vi "BestYForAnyElements.vi"(8 "inimigos":bool=TRUE, 9 "Position to be analyzed":dbl[](array[numeric]), 10 "Game":refnum<class "Game.lvclass">, 11 "Utilities in":refnum<class "Utilities.lvclass">) -> (2 "Goal Gap":dbl, 3 "Utilities out":refnum<class "Utilities.lvclass">)   [LabVIEW 2023, in "Utilities.lvclass"]
uses:
  Utilities.lvclass
  segment.ctl
  Game_class/Game.lvclass
  Vision_class/Old vision/SSL Detection Frame Simple Estimator Cameras VelCmd Folder/Core/AI Ball.ctl
  pos.ctl
  Game_class/Game.lvclass/Game.ctl
  Team_class/Team.lvclass/Team.ctl
  Object_class/Object.lvclass/Object.ctl
  Object_class/Read x.vi
  Object_class/Read y.vi
  <vilib>/Analysis/baseanly.llb/Real Dot Product.vi
  Game_class/Read FieldRef.vi
  Game_class/Read EnemyRef.vi
  Game_class/Read AllyRef.vi
  Team_class/Read RobotRef.vi
  Ally_class/Ally.lvclass
  C:/Users/roboi/Downloads/VSS_AI-Larc2023 - Copia (2)/Team_class/Team.lvclass
  Enemy_class/Enemy.lvclass
  Robot_class/Robot.lvclass
  C:/Users/roboi/Downloads/VSS_AI-Larc2023 - Copia (2)/Object_class/Object.lvclass
  Field_class/Field.lvclass
  <vilib>/Analysis/NI_AALBase.lvlib
panel:
  out "Best y":dbl
  out "Gap Coord":dbl[](array[numeric])
  in  "eclipse angle eps":dbl=0.035 format="%#_13g"
  out "Eclipse":bool
  out "Vetor de segmentos (sombras)":T1[](array[typedef])
  out "Vetor de segmentos ordenado":T1[](array[typedef])
  out "pilha output (merged)":T1[](array[typedef])
  in  "Maior intervalo":bool
  out "Vetor de gaps":T1[](array[typedef])
  in  "Best y para varredura?":bool
  in  "Ball false":dbl[](array[numeric])
  out "Vetor de gaps \ncorreto":T1[](array[typedef])
  out "error out":errorcluster
  in  "error in (no error)":errorcluster
types:
  T1 = typedef "Utilities.lvclass/segment.ctl" = cluster{"up":dbl, "down":dbl}
  T2 = typedef "pos.ctl" = cluster{"x":dbl, "y":dbl}
  T3 = typedef "AI Ball.ctl" = cluster{"x":dbl, "y":dbl, "timestamp":timestamp, "Vel_x":dbl, "Vel_y":dbl, "Pos Bola Est":dbl[], "Valid":bool}
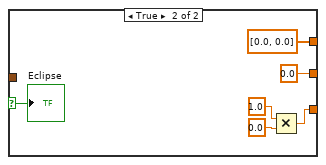
[diagram p4: hidden frame]
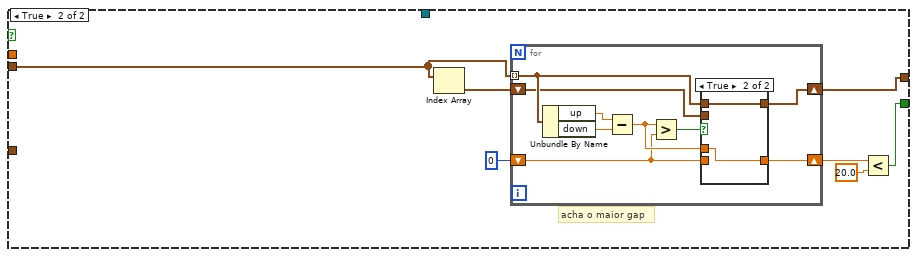
[diagram p7: hidden frame]
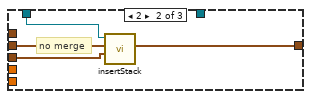
[diagram p9: hidden frame]
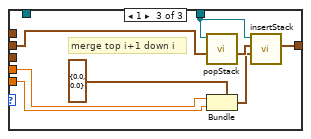
[diagram p10: hidden frame]
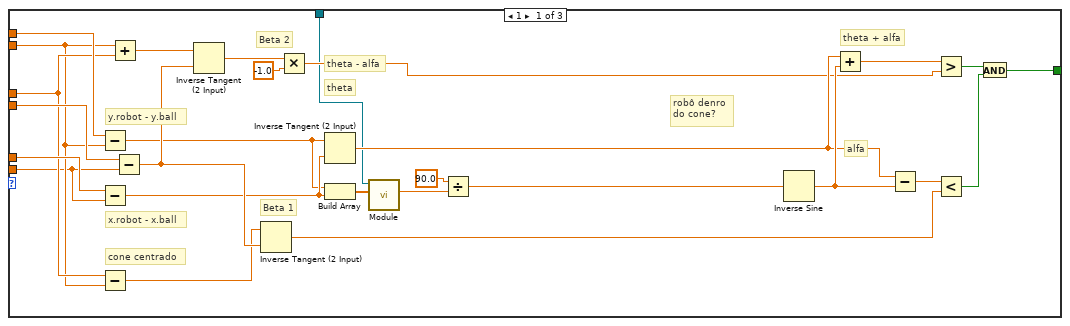
[diagram p12: hidden frame]
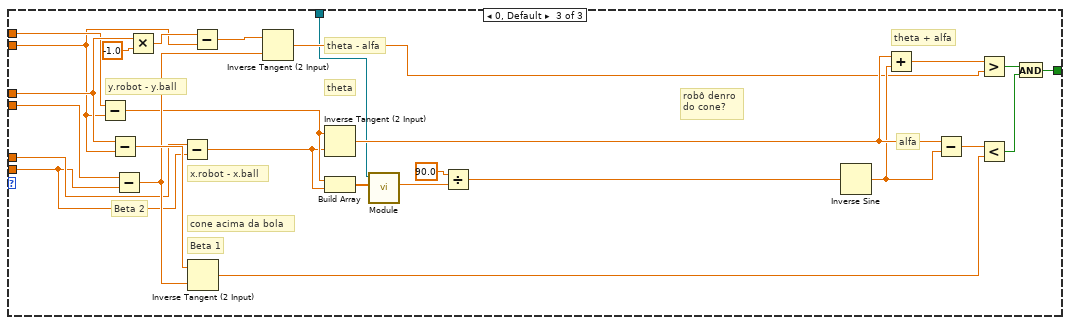
[diagram p13: hidden frame]
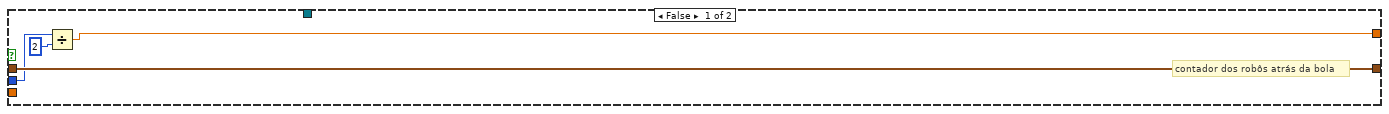
[diagram p14: hidden frame]
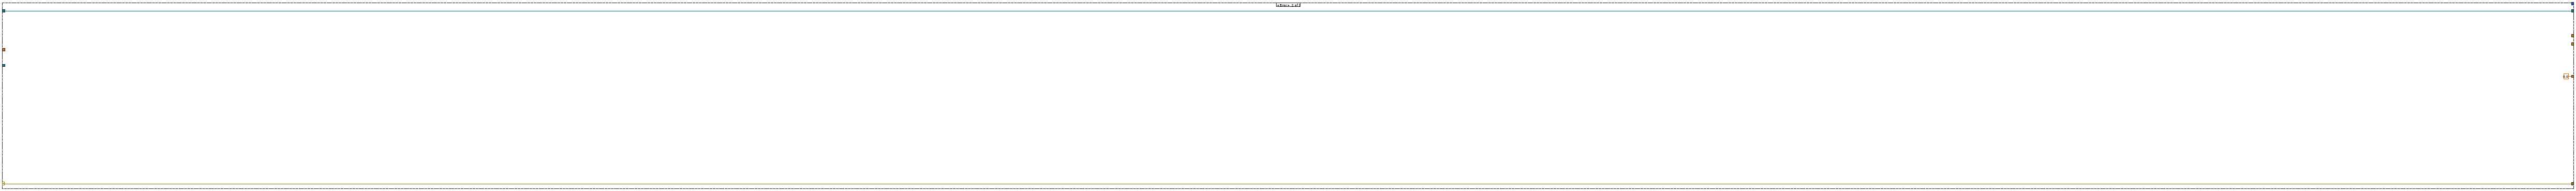
[diagram p16: hidden frame]
diagram:
  # "Gap kick is now a value from 0 to 1\n0 -> goal not free\n1 - > goal totally free"
  n1 = case shown="No Error" "error in (no error)" {
    selector: "error in (no error)" -> [w64 w427]
    tunnel: [w64 w427] -> w10
    tunnel: [w17 w426] -> w8
    tunnel: "Utilities in" -> [w17 w426]
    tunnel: "Game" -> [w29 _]
    tunnel: [w28 _] -> w6
    tunnel: [w27 _] -> w2
    tunnel: [w26 0.0] -> w5
    tunnel: [w16 _] -> w3
    tunnel: "Position to be analyzed" -> [w15 _]
    frame No Error {
      w42 = T3 {"x"=0.0, "y"=0.0, "timestamp"=timestamp(0 s since 1904-01-01), "Vel_x"=0.0, "Vel_y"=0.0, "Pos Bola Est"=[], "Valid"=FALSE} ("element")
      # "goal_width/2"
      # "field_length/2"
      # "balls"
      # "vetor de gaps"
      # "upper"
      n2 = property class="Game"(reference=w29) -> ("FieldRef"=w24:refnum<class "Field.lvclass">, "EnemyRef"=w21:refnum<class "Enemy.lvclass">, "AllyRef"=w19:refnum<class "Ally.lvclass">)  [unwired: 1 in, 2 out]
      n3 = property class="Enemy"(reference=w21) -> ("RobotRef"=w20:refnum<class "Robot.lvclass">[])  [unwired: 1 in, 2 out]
      n4 = property class="Ally"(reference=w19) -> ("RobotRef"=w18:refnum<class "Robot.lvclass">[])  [unwired: 1 in, 2 out]
      n5 = Index Array(array=w15) -> (element #1=w14:dbl, element #2=w13:dbl)  [unwired: 2 in]
      n6 = property class="Field"(reference=w24) -> ("field_length"=w22:i32, "goal_width"=w16:i32)  [unwired: 1 in, 2 out]
      n7 = Bundle By Name(cluster=T2 {"x"=0.0, "y"=0.0} ("pos"), "x"=w14, "y"=w13) -> (w23:T2)
      n8 = Select(t=w20, s="inimigos", f=w18) -> (s? t:f=w46:refnum<class "Robot.lvclass">[])
      n9 = Index Array(array="Ball false") -> (element #1=w45:dbl, element #2=w44:dbl)  [unwired: 2 in]
      n10 = Bundle By Name(cluster=w42, "x"=w45, "y"=w44) -> ()  [unwired: 1 out]
      n11 = case shown="False" "Best y para varredura?" {
        tunnel: [w119 w120] -> w41
        tunnel: w23 -> [w119 w120]
        tunnel: w42 -> [_ _]
        frame False {
        }
        frame True {
        }
      }
      n12 = Divide(x=w16, y=u32 2 ("x")) -> (x/y=w34:dbl)
      n13 = for {
        shift-right: [w268] -> w49
        shift-left: T1[] [] -> [w267]
        tunnel: w22 -> [w245]
        tunnel: w34 -> [w247]
        tunnel: w34 -> [w265]
        shift-right: [w264] -> w47
        shift-left: _ -> [_]
        tunnel: w46 -> [w237] mode=indexing
        tunnel: "inimigos" -> [w262]
        tunnel: w41 -> [w241]
        tunnel: w17 -> [w234]
        tunnel: w17 -> [w233]
        # "y ball"
        # "x ball"
        # "y.robot"
        # "x.robot"
        # "field_length/2"
        # "goal_width/2"
        # "y ball"
        # "x ball"
        n14 = property class="Robot"(reference=w237) -> ("x"=w236:dbl, "y"=w235:dbl)  [unwired: 1 in, 2 out]
        n15 = Unbundle By Name(w241) -> ("x"=w240:dbl, "y"=w238:dbl)
        n16 = Divide(x=w245, y=2.0) -> (x/y=w244:dbl)
        n17 = Multiply(x=w247, y=-1.0) -> (x*y=w251:dbl)
        n18 = Greater?(x=w238, y=w247) -> (0:w250:bool)
        n19 = Less?(x=w238, y=w251) -> (x < y?=w249:bool)
        n20 = Absolute Value(x=w240) -> (abs(x)=w260:dbl)
        n21 = Absolute Value(x=w236) -> (abs(x)=w266:dbl)
        n22 = Multiply(x=w236, y=-1.0) -> (x*y=w261:dbl)
        n23 = Greater?(x=w266, y=w260) -> (0:w259:bool)
        n24 = Select(t=w236, s=w262, f=w261) -> (s? t:f=w242:dbl)
        n25 = Select(t=1, s=w250, f=0) -> (s? t:f=w257:i32)
        n26 = Select(t=0, s=w249, f=1) -> (s? t:f=w258:i32)
        n27 = Add(x=w257, y=w258) -> (x+y=w248:i32)
        n28 = case shown="2" w248 {
          tunnel: w247 -> [w272 w299 w348]
          tunnel: w244 -> [w293 w319 w350]
          tunnel: w242 -> [w280 w306 w343]
          tunnel: w235 -> [w279 w307 w344]
          tunnel: [w281 w308 w334] -> w239
          tunnel: w240 -> [w270 w297 w326]
          tunnel: w238 -> [w271 w298 w327]
          tunnel: w234 -> [w269 w296 w325]
          frame 1 {
            # "robô denro\ndo cone?"
            # "cone centrado"
            # "theta - alfa"
            # "theta + alfa"
            # "theta"
            # "alfa"
            # "x.robot - x.ball"
            # "y.robot - y.ball"
            # "Beta 2"
            # "Beta 1"
            n29 = Subtract(x=w279, y=w271) -> (x-y=w282:dbl)
            n30 = Subtract(x=w280, y=w270) -> (x-y=w283:dbl)
            n31 = Subtract(x=w272, y=w271) -> (x-y=w294:dbl)
            n32 = Add(x=w271, y=w272) -> (x+y=w292:dbl)
            n33 = Subtract(x=w293, y=w270) -> (x-y=w295:dbl)
            n34 = Inverse Tangent (2 Input)(1:w295, 2:w292) -> (0:w291:dbl)
            n35 = Inverse Tangent (2 Input)(1:w295, 2:w294) -> (0:w275:dbl)
            n36 = Multiply(x=w291, y=-1.0) -> (x*y=w277:dbl)
            n37 = Inverse Tangent (2 Input)(1:w283, 2:w282) -> (0:w288:dbl)
            n38 = Build Array(w282, w283) -> (w284:dbl[])
            n39 = call "Module.vi"("2D vector"=w284, "Utilities in"=w269) -> ("Modulo"=w285:dbl)  [unwired: 7 in, 2 out]
            n40 = Divide(x=90.0, y=w285) -> (x/y=w286:dbl)
            n41 = Inverse Sine(1:w286) -> (0:w289:dbl)
            n42 = Add(x=w288, y=w289) -> (x+y=w278:dbl)
            n43 = Subtract(x=w288, y=w289) -> (x-y=w276:dbl)
            n44 = Greater?(x=w278, y=w277) -> (0:w273:bool)
            n45 = Less?(x=w276, y=w275) -> (x < y?=w274:bool)
            n46 = And(x=w273, y=w274) -> (x .and. y?=w281:bool)
          }
          frame 2 {
            # "robô denro\ndo cone?"
            # "cone abaixo da bola"
            # "theta - alfa"
            # "theta + alfa"
            # "theta"
            # "alfa"
            # "x.robot - x.ball"
            # "y.robot - y.ball"
            # "Beta 2"
            # "Beta 1"
            n47 = Add(x=w298, y=w299) -> (x+y=w322:dbl)
            n48 = Subtract(x=w298, y=w299) -> (x-y=w321:dbl)
            n49 = Subtract(x=w319, y=w297) -> (x-y=w320:dbl)
            n50 = Inverse Tangent (2 Input)(1:w320, 2:w321) -> (0:w317:dbl)
            n51 = Inverse Tangent (2 Input)(1:w320, 2:w322) -> (0:w323:dbl)
            n52 = Subtract(x=w307, y=w298) -> (x-y=w309:dbl)
            n53 = Multiply(x=w323, y=-1.0) -> (x*y=w304:dbl)
            n54 = Subtract(x=w306, y=w297) -> (x-y=w310:dbl)
            n55 = Inverse Tangent (2 Input)(1:w310, 2:w309) -> (0:w315:dbl)
            n56 = Build Array(w309, w310) -> (w311:dbl[])
            n57 = call "Module.vi"("2D vector"=w311, "Utilities in"=w296) -> ("Modulo"=w312:dbl)  [unwired: 7 in, 2 out]
            n58 = Multiply(x=w317, y=-1.0) -> (x*y=w302:dbl)
            n59 = Divide(x=90.0, y=w312) -> (x/y=w313:dbl)
            n60 = Inverse Sine(1:w313) -> (0:w316:dbl)
            n61 = Add(x=w315, y=w316) -> (x+y=w305:dbl)
            n62 = Subtract(x=w315, y=w316) -> (x-y=w303:dbl)
            n63 = Less?(x=w303, y=w302) -> (x < y?=w301:bool)
            n64 = Greater?(x=w305, y=w304) -> (0:w300:bool)
            n65 = And(x=w300, y=w301) -> (x .and. y?=w308:bool)
          }
          frame 0, Default {
            # "robô denro\ndo cone?"
            # "cone acima da bola"
            # "theta - alfa"
            # "theta + alfa"
            # "theta"
            # "alfa"
            # "x.robot - x.ball"
            # "y.robot - y.ball"
            # "Beta 2"
            # "Beta 1"
            n66 = Subtract(x=w344, y=w327) -> (x-y=w342:dbl)
            n67 = Subtract(x=w348, y=w327) -> (x-y=w351:dbl)
            n68 = Subtract(x=w350, y=w326) -> (x-y=w345:dbl)
            n69 = Multiply(x=w348, y=-1.0) -> (x*y=w347:dbl)
            n70 = Subtract(x=w343, y=w326) -> (x-y=w341:dbl)
            n71 = Inverse Tangent (2 Input)(1:w345, 2:w351) -> (0:w329:dbl)
            n72 = Subtract(x=w347, y=w327) -> (x-y=w346:dbl)
            n73 = Inverse Tangent (2 Input)(1:w345, 2:w346) -> (0:w332:dbl)
            n74 = Inverse Tangent (2 Input)(1:w341, 2:w342) -> (0:w336:dbl)
            n75 = Build Array(w342, w341) -> (w340:dbl[])
            n76 = call "Module.vi"("2D vector"=w340, "Utilities in"=w325) -> ("Modulo"=w339:dbl)  [unwired: 7 in, 2 out]
            n77 = Divide(x=90.0, y=w339) -> (x/y=w338:dbl)
            n78 = Inverse Sine(1:w338) -> (0:w335:dbl)
            n79 = Add(x=w336, y=w335) -> (x+y=w333:dbl)
            n80 = Subtract(x=w336, y=w335) -> (x-y=w330:dbl)
            n81 = Greater?(x=w333, y=w332) -> (0:w331:bool)
            n82 = Less?(x=w330, y=w329) -> (x < y?=w328:bool)
            n83 = And(x=w331, y=w328) -> (x .and. y?=w334:bool)
          }
        }
        n84 = And(x=w259, y=w239) -> (x .and. y?=w243:bool)
        n85 = case shown="True" w243 {
          tunnel: [w355 w363] -> w268
          tunnel: w267 -> [w355 w365]
          tunnel: w245 -> [w354 w370]
          tunnel: w247 -> [_ w369]
          tunnel: w265 -> [_ w362]
          tunnel: [w352 w361] -> w264
          tunnel: w235 -> [_ w360]
          tunnel: w242 -> [_ w359]
          tunnel: w240 -> [_ w357]
          tunnel: w238 -> [_ w358]
          tunnel: w233 -> [_ w356]
          frame False {
            # "contador dos robôs atrás da bola"
            n86 = Divide(x=w354, y=u32 2) -> (x/y=w352:dbl)
          }
          frame True {
            n87 = flat-sequence {
              tunnel: w360 -> [w406]
              tunnel: w370 -> [w402]
              tunnel: w369 -> [w387]
              tunnel: [w377] -> w368
              tunnel: [w376] -> w367
              tunnel: [w388] -> w366
              tunnel: w365 -> [w381]
              tunnel: [w381] -> w364
              tunnel: [w375] -> w361
              tunnel: w359 -> [w374]
              tunnel: w358 -> [w372]
              tunnel: w357 -> [w373]
              tunnel: w356 -> [w371]
              tunnel: w368 -> [w410]
              tunnel: w367 -> [w409]
              tunnel: w366 -> [w411]
              tunnel: w364 -> [w412]
              tunnel: [w408] -> w363
              tunnel: w362 -> [w407]
              frame #0 {
                # "theta - alfa"
                # "alfa + theta"
                # "theta"
                # "alfa"
                # "x.robot - x.ball"
                # "y.robot - y.ball"
                n88 = Subtract(x=w406, y=w372) -> (x-y=w386:dbl)
                n89 = Subtract(x=w374, y=w373) -> (x-y=w385:dbl)
                n90 = Inverse Tangent (2 Input)(1:w385, 2:w386) -> (0:w384:dbl)
                n91 = Build Array(w386, w385) -> (w405:dbl[])
                n92 = call "Module.vi"("2D vector"=w405, "Utilities in"=w371) -> ("Modulo"=w403:dbl)  [unwired: 7 in, 2 out]
                n93 = Divide(x=90.0, y=w403) -> (x/y=w383:dbl)
                n94 = Inverse Sine(1:w383) -> (0:w382:dbl)
                n95 = Add(x=w384, y=w382) -> (x+y=w400:dbl)
                n96 = Subtract(x=w384, y=w382) -> (x-y=w398:dbl)
                n97 = Divide(x=w402, y=u32 2 ("x")) -> (x/y=w375:dbl)
                n98 = Subtract(x=w375, y=w373) -> (x-y=w378:dbl)
                n99 = Tangent(1:w398) -> (0:w397:dbl)
                n100 = Multiply(x=w397, y=w378) -> (x*y=w379:dbl)
                n101 = Tangent(1:w400) -> (0:w399:dbl)
                n102 = Multiply(x=w399, y=w378) -> (x*y=w380:dbl)
                n103 = Add(x=w379, y=w372) -> (x+y=w376:dbl)
                n104 = Multiply(x=w387, y=-1.0) -> (x*y=w393:dbl)
                n105 = Add(x=w380, y=w372) -> (x+y=w377:dbl)
                n106 = Greater?(x=w376, y=w387) -> (0:w395:bool)
                n107 = Less?(x=w376, y=w393) -> (x < y?=w391:bool)
                n108 = Greater?(x=w377, y=w387) -> (0:w396:bool)
                n109 = Less?(x=w377, y=w393) -> (x < y?=w392:bool)
                n110 = And(x=w396, y=w395) -> (x .and. y?=w390:bool)
                n111 = And(x=w392, y=w391) -> (x .and. y?=w389:bool)
                n112 = Or(x=w390, y=w389) -> (x .or. y?=w388:bool)
              }
              frame #1 {
                # "goal_width/2"
                n113 = case shown="False" w411 {
                  tunnel: [w421 w424] -> w408
                  tunnel: w412 -> [w420 w424]
                  tunnel: w410 -> [w419 _]
                  tunnel: w409 -> [w417 _]
                  tunnel: w407 -> [w416 _]
                  frame False {
                    n114 = Max & Min(x=w419, y=w416) -> (min(x,y)=w418:dbl)  [unwired: 1 out]
                    n115 = Multiply(x=w416, y=-1.0) -> (x*y=w414:dbl)
                    n116 = Max & Min(x=w417, y=w414) -> (max(x,y)=w413:dbl)  [unwired: 1 out]
                    n117 = Bundle(cluster=T1 {"up"=0.0, "down"=0.0} ("segment 2"), "up"=w418, "down"=w413) -> (w422:T1)
                    n118 = Insert Into Array(array=w420, new element=w422) -> (w421:T1[])  [unwired: 1 in]
                  }
                  frame True {
                  }
                }
              }
            }
          }
        }
      }
      "Vetor de segmentos (sombras)" <- w49
      n119 = Multiply(x=w34, y=-1.0) -> (x*y=w50:dbl)
      n120 = Sort 1D Array(array=w49) -> (sorted array=w61:T1[])
      "Vetor de segmentos ordenado" <- w61
      n121 = Index Array(array=w61) -> (element=w60:T1)  [unwired: 1 in]
      n122 = call-dynamic "insertStack.vi"("novo elemento"=w60, "pilha input"=T1[] [], "Utilities in"=w17) -> ("pilha output"=w58:T1[])  [unwired: 5 in, 2 out]
      n123 = for {
        shift-right: [w191] -> w57
        shift-left: w58 -> [w193]
        tunnel: w61 -> [w192] mode=indexing
        tunnel: w17 -> [w190]
        tunnel: w17 -> [w189]
        tunnel: w17 -> [w188]
        i -> [w194]
        n124 = case shown="Default" w194 {
          tunnel: w193 -> [w201 w232]
          tunnel: w192 -> [w204 _]
          tunnel: [w202 w232] -> w191
          tunnel: w190 -> [w197 _]
          tunnel: w189 -> [w196 _]
          tunnel: w188 -> [w195 _]
          frame Default {
            # "pilha"
            # "i+1"
            # "i"
            # "i+1"
            # "i"
            n125 = Unbundle By Name(w204) -> ("down"=w199:dbl, "up"=w206:dbl)
            n126 = call-dynamic "topStack.vi"("pilha input"=w201, "Utilities in"=w195) -> ("top"=w203:T1)  [unwired: 7 in, 2 out]
            n127 = Unbundle By Name(w203) -> ("up"=w200:dbl, "down"=w205:dbl)
            n128 = Greater Or Equal?(x=w199, y=w200) -> (x >= y?=w198:bool)
            n129 = Less?(x=w199, y=w205) -> (x < y?=w208:bool)
            n130 = Select(t=1, s=w198, f=0) -> (s? t:f=w210:i32)
            n131 = Select(t=0, s=w208, f=1) -> (s? t:f=w209:i32)
            n132 = Add(x=w210, y=w209) -> (x+y=w207:i32)
            n133 = case shown="0, Default" w207 {
              tunnel: w206 -> [_ _ w230]
              tunnel: w205 -> [_ _ w229]
              tunnel: w203 -> [_ _ _]
              tunnel: w204 -> [w216 w222 _]
              tunnel: [w219 w221 w225] -> w202
              tunnel: w201 -> [w218 w223 w228]
              tunnel: w197 -> [w215 w220 _]
              tunnel: w196 -> [_ _ w224]
              frame 0, Default {
                # "merge:  i+1"
                n134 = call-dynamic "popStack.vi"("pilha input"=w218, "Utilities in"=w215) -> ("pilha output"=w217:T1[])  [unwired: 7 in, 2 out]
                n135 = call-dynamic "insertStack.vi"("novo elemento"=w216, "pilha input"=w217, "Utilities in"=w215) -> ("pilha output"=w219:T1[])  [unwired: 5 in, 2 out]
              }
              frame 2 {
                # "no merge"
                n136 = call-dynamic "insertStack.vi"("novo elemento"=w222, "pilha input"=w223, "Utilities in"=w220) -> ("pilha output"=w221:T1[])  [unwired: 5 in, 2 out]
              }
              frame 1 {
                # "merge top i+1 down i"
                n137 = call-dynamic "popStack.vi"("pilha input"=w228, "Utilities in"=w224) -> ("pilha output"=w227:T1[])  [unwired: 7 in, 2 out]
                n138 = Bundle(cluster=T1 {"up"=0.0, "down"=0.0} ("segment 2"), "up"=w230, "down"=w229) -> (w226:T1)
                n139 = call-dynamic "insertStack.vi"("novo elemento"=w226, "pilha input"=w227, "Utilities in"=w224) -> ("pilha output"=w225:T1[])  [unwired: 5 in, 2 out]
              }
            }
          }
          frame 0 {
          }
        }
      }
      "pilha output (merged)" <- w57
      n140 = Reverse 1D Array(array=w57) -> (reversed array=w56:T1[])
      n141 = for {
        tunnel: w56 -> [w187] mode=indexing
        shift-right: [w181] -> w53
        shift-left: T1[] [] -> [w183]
        shift-right: [w182] -> w52
        shift-left: w34 -> [w184]
        n142 = Unbundle By Name(w187) -> ("up"=w180:dbl, "down"=w182:dbl)
        n143 = Bundle(cluster=T1 {"up"=0.0, "down"=0.0} ("segment 2"), "up"=w184, "down"=w180) -> (w186:T1)
        n144 = Insert Into Array(array=w183, new element=w186) -> (w181:T1[])  [unwired: 1 in]
      }
      n145 = Bundle(cluster=T1 {"up"=0.0, "down"=0.0} ("segment 2"), "up"=w52, "down"=w50) -> (w55:T1)
      n146 = Insert Into Array(array=w53, new element=w55) -> (w35:T1[])  [unwired: 1 in]
      n147 = Array Size(array=w35) -> (size(s)=w37:i32)
      n148 = Decrement(x=w37) -> (x-1=w36:i32)
      n149 = for {
        N: w36 -> [_]
        shift-right: [w83] -> w33
        shift-left: w35 -> [w85]
        i -> [w84]
        n150 = Increment(x=w84) -> (x+1=w93:i32)
        n151 = Index Array(array=w85, index=w84) -> (element=w86:T1)
        n152 = Index Array(array=w85, index=w93) -> (element=w92:T1)
        n153 = Unbundle By Name(w86) -> ("up"=w88:dbl, "down"=w91:dbl)
        n154 = Unbundle By Name(w92) -> ("up"=w90:dbl, "down"=w87:dbl)
        n155 = Equal?(x=w91, y=w90) -> (x = y?=w89:bool)
        n156 = case shown="True" w89 {
          tunnel: w88 -> [_ w103]
          tunnel: w87 -> [_ w102]
          tunnel: w86 -> [_ w101]
          tunnel: w85 -> [w94 w99]
          tunnel: w84 -> [_ w96]
          tunnel: [w94 w95] -> w83
          frame False {
          }
          frame True {
            n157 = Bundle By Name(cluster=w101, "up"=w103, "down"=w102) -> (w97:T1)
            n158 = Delete From Array(array=w99, length=2, index=w96) -> (array with subset deleted=w98:T1[])  [unwired: 1 out]
            n159 = Insert Into Array(array=w98, index=w96, new element=w97) -> (w95:T1[])
          }
        }
      }
      "Vetor de gaps" <- w33
      n160 = for {
        tunnel: w34 -> [w74]
        tunnel: w33 -> [w67] mode=indexing
        shift-right: [w69] -> w30
        shift-left: T1[] [] -> [w68]
        n161 = Unbundle By Name(w67) -> ("up"=w66:dbl, "down"=w65:dbl)
        n162 = Multiply(x=w74, y=-1.0) -> (x*y=w73:dbl)
        n163 = Greater?(x=w66, y=w74) -> (0:w71:bool)
        n164 = Less?(x=w65, y=w73) -> (x < y?=w70:bool)
        n165 = Or(x=w71, y=w70) -> (x .or. y?=w72:bool)
        n166 = case shown="False" w72 {
          tunnel: [w76 w79] -> w69
          tunnel: w68 -> [w76 w80]
          tunnel: w66 -> [_ w77]
          tunnel: w65 -> [_ w78]
          frame True {
          }
          frame False {
            n167 = Bundle(cluster=T1 {"up"=0.0, "down"=0.0} ("segment 2"), "up"=w77, "down"=w78) -> (w81:T1)
            n168 = Insert Into Array(array=w80, new element=w81) -> (w79:T1[])  [unwired: 1 in]
          }
        }
      }
      "Vetor de gaps \ncorreto" <- w30
      n169 = case shown="False" "Maior intervalo" {
        tunnel: [w124 w163] -> w38
        tunnel: [w123 w161] -> w39
        tunnel: w30 -> [w130 w162]
        tunnel: w41 -> [w122 _]
        tunnel: w47 -> [w127 _]
        tunnel: w17 -> [w121 _]
        frame False {
          # "acha o maior ângulo"
          n170 = Index Array(array=w130) -> (element=w131:T1)  [unwired: 1 in]
          n171 = Unbundle By Name(w122) -> ("x"=w129:dbl, "y"=w128:dbl)
          n172 = for {
            tunnel: w130 -> [w153] mode=indexing
            shift-right: [w154] -> w126
            shift-left: 0 -> [w136]
            shift-right: [w152] -> w123
            shift-left: w131 -> [w151]
            tunnel: w129 -> [w135]
            tunnel: w128 -> [w134]
            tunnel: w127 -> [w150]
            tunnel: w121 -> [w133]
            # "theta"
            # "cos (theta)"
            # "vetor bola-down"
            # "vetor bola-up"
            n173 = Unbundle By Name(w153) -> ("up"=w149:dbl, "down"=w146:dbl)
            n174 = Subtract(x=w150, y=w135) -> (x-y=w147:dbl)
            n175 = Subtract(x=w149, y=w134) -> (x-y=w148:dbl)
            n176 = Subtract(x=w146, y=w134) -> (x-y=w145:dbl)
            n177 = Build Array(w147, w145) -> (w143:dbl[])
            n178 = Build Array(w147, w148) -> (w144:dbl[])
            n179 = call "Module.vi"("2D vector"=w144, "Utilities in"=w133) -> ("Modulo"=w142:dbl)  [unwired: 7 in, 2 out]
            n180 = call-poly <vilib>:"Dot Product.vi"("Y Vector"=w143, "X Vector"=w144) -> ("X * Y"=w140:dbl)  [unwired: 1 out]
            n181 = call "Module.vi"("2D vector"=w143, "Utilities in"=w133) -> ("Modulo"=w141:dbl)  [unwired: 7 in, 2 out]
            n182 = Multiply(x=w142, y=w141) -> (x*y=w139:dbl)
            n183 = Divide(x=w140, y=w139) -> (x/y=w138:dbl)
            n184 = Inverse Cosine(1:w138) -> (0:w137:dbl)
            n185 = Greater?(x=w137, y=w136) -> (0:w155:bool)
            n186 = case shown="True" w155 {
              tunnel: w137 -> [_ w159]
              tunnel: [w156 w159] -> w154
              tunnel: w153 -> [_ w158]
              tunnel: [w157 w158] -> w152
              tunnel: w151 -> [w157 _]
              tunnel: w136 -> [w156 _]
              frame False {
              }
              frame True {
              }
            }
          }
          n187 = Less?(x=w126, y="eclipse angle eps") -> (x < y?=w124:bool)
        }
        frame True {
          # "acha o maior gap"
          n188 = Index Array(array=w162) -> (element=w165:T1)  [unwired: 1 in]
          n189 = for {
            tunnel: w162 -> [w170] mode=indexing
            shift-right: [w171] -> w164
            shift-left: 0 -> [w168]
            shift-right: [w169] -> w161
            shift-left: w165 -> [w167]
            n190 = Unbundle By Name(w170) -> ("up"=w175:dbl, "down"=w174:dbl)
            n191 = Subtract(x=w175, y=w174) -> (x-y=w172:dbl)
            n192 = Greater?(x=w172, y=w168) -> (0:w173:bool)
            n193 = case shown="True" w173 {
              tunnel: w172 -> [_ w179]
              tunnel: [w177 w179] -> w171
              tunnel: w170 -> [_ w178]
              tunnel: [w176 w178] -> w169
              tunnel: w168 -> [w177 _]
              tunnel: w167 -> [w176 _]
              frame False {
              }
              frame True {
              }
            }
          }
          n194 = Less?(x=w164, y=20.0) -> (x < y?=w163:bool)
        }
      }
      n195 = case shown="False" w38 {
        selector: w38 -> [_ w118]
        tunnel: w39 -> [w110 _]
        tunnel: [w109 w115] -> w26
        tunnel: [w107 0.0] -> w27
        tunnel: [w104 dbl[] [0.0, 0.0] ("Gap Coord")] -> w28
        frame False {
          n196 = Unbundle By Name(w110) -> ("up"=w106:dbl, "down"=w105:dbl)
          n197 = Subtract(x=w106, y=w105) -> (x-y=w108:dbl)
          n198 = Add(x=w106, y=w105) -> (x+y=w111:dbl)
          n199 = Build Array(w106, w105) -> (w104:dbl[])
          n200 = Absolute Value(x=w108) -> (abs(x)=w107:dbl)
          n201 = Divide(x=w111, y=2.0) -> (x/y=w109:dbl)
        }
        frame True {
          n202 = Multiply(x=1.0, y=0.0) -> (x*y=w115:dbl)
          "Eclipse" <- w118
        }
      }
    }
    frame Error {
    }
  }
  "error out" <- w10
  "Utilities out" <- w8
  "Gap Coord" <- w6
  "Best y" <- w5
  n203 = Divide(x=w2, y=w3) -> (x/y=→"Goal Gap":dbl)
